vi "DSF.Engine.Interface.Set Error Queue.vi"(10 "Error Queue":T1, 11 "Interface in":refnum<class "DSF.Engine.Interface.lvclass">) -> (3 "Interface out":refnum<class "DSF.Engine.Interface.lvclass">)   [LabVIEW 2017, in "Data Sharing Framework Engine.lvlib" / "DSF.Engine.Interface.lvclass"]
uses:
  DSF.Engine.Interface.lvclass
  DSF.Engine.Interface.Error Queue.Ref.ctl
  DSF.Engine.Interface.lvclass/DSF.Engine.Interface.ctl
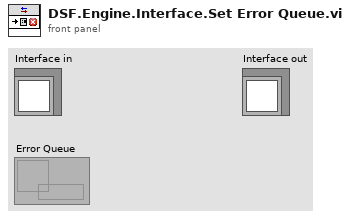
[diagram p1: front panel]
types:
  T1 = typedef "Data Sharing Framework Engine.lvlib/DSF.Engine.Interface.lvclass/DSF.Engine.Interface.Error Queue.Ref.ctl" = refnum<queue>
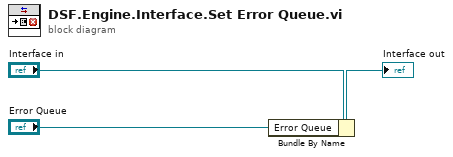
[diagram p0: block diagram]
diagram:
  n1 = Bundle By Name(cluster="Interface in", "Error Queue"="Error Queue") -> (→"Interface out":refnum<class "DSF.Engine.Interface.lvclass">)
